vi "Save Model.vi"(7 "Group name":string, 8 "error in (no error)":errorcluster, 9 "Input onfiguration":T1={"Input File Path"=path "", "from scan..."=0, "...to scan"=0, "Lead resistance"=0.0, "Correct conductance "=FALSE, "Model parameters gap 1"={"Delta 1"=0.0, "Delta 2"=0.0, "Gama"=0.0, "Z"=0.0, "P"=0.0, "T"=0.0, "Integration range"=0.0, "Resolution"=0.0}, "Scale"=0.0, "Offset"=0.0, "Append channels"=[], "Model parameters gap 2"={"Delta 1"=0.0, "Delta 2"=0.0, "Gama"=0.0, "Z"=0.0, "P"=0.0, "T"=0.0, "Integration range"=0.0, "Resolution"=0.0}, "Gap 2 weight"=0.0, "Background conductance"=0.0, "Channels"=["V", "I", "dIdV"], "Preserve model history"=FALSE, "dIdV units"=enum."S"} {"Background conductance" step=0.0001 format="%#_6pS"; "Model parameters gap 2"."Delta 1" step=0.001 format="%#_6peV"; "Model parameters gap 2"."Resolution" format="%#_6peV"; "Model parameters gap 2"."Integration range" format="%#_6peV"; "Model parameters gap 2"."T" format="%#_6pK"; "Model parameters gap 2"."Delta 2" step=0.001 format="%#_6peV"; "Model parameters gap 2"."Gama" step=0.001 format="%#_6peV"; "Offset" scale=0.0..0.1; "Scale" scale=0.0..0.03; "Model parameters gap 1"."Delta 1" step=0.001 format="%#_6peV"; "Model parameters gap 1"."Resolution" format="%#_6peV"; "Model parameters gap 1"."Integration range" format="%#_6peV"; "Model parameters gap 1"."T" format="%#_6pK"; "Model parameters gap 1"."Delta 2" step=0.001 format="%#_6peV"; "Model parameters gap 1"."Gama" step=0.001 format="%#_6peV"; "Lead resistance" scale=0.0..80.0}, 10 "Save File Path":path, 11 "Point Contact Model in":refnum<class "Point Contact Model.lvclass">) -> (0 "error out":errorcluster, 1 "output group":string, 2 "Save File Path out":path, 3 "Point Contact Model out":refnum<class "Point Contact Model.lvclass">)   [LabVIEW 2021, in "Point Contact Model.lvclass"]
uses:
  Point Contact Model.lvclass
  Controls/PCS Config.ctl
  Parameters.ctl
  Point Contact Model.lvclass/Point Contact Model.ctl
panel:
  # "V"
  # "I"
  # "dIdV"
  # "<="
  # "<="
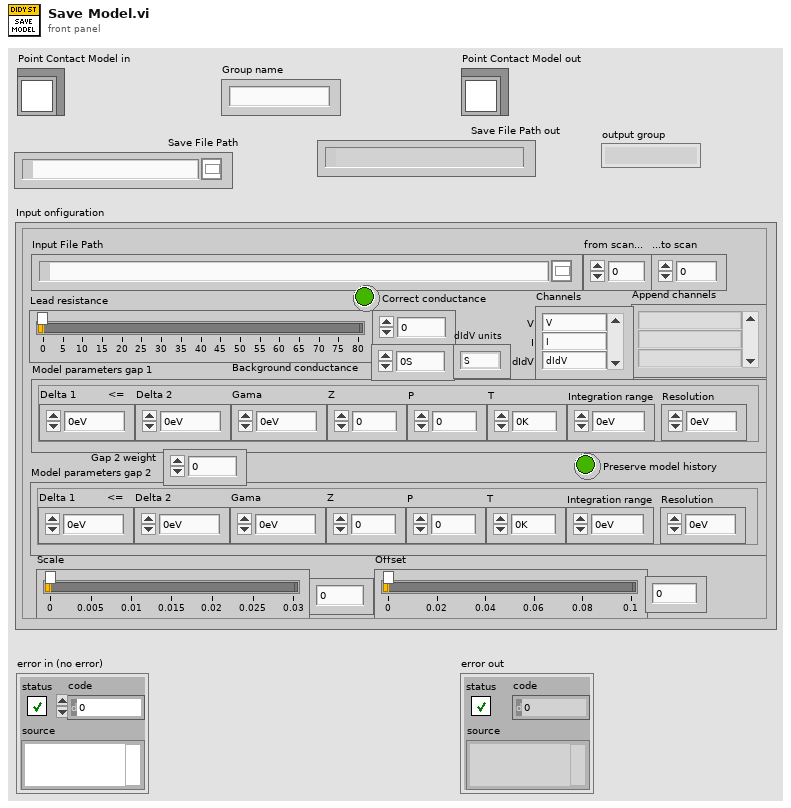
[diagram p1: front panel]
types:
  T1 = typedef "PCS Config.ctl" = cluster{"Input File Path":path, "from scan...":i32, "...to scan":i32, "Lead resistance":dbl, "Correct conductance ":bool, "Model parameters gap 1":T2, "Scale":dbl, "Offset":dbl, "Append channels":string[], "Model parameters gap 2":T2, "Gap 2 weight":dbl, "Background conductance":dbl, "Channels":string[], "Preserve model history":bool, "dIdV units":enum16{"S", "Ohm", "V"}}
  T2 = typedef "Parameters.ctl" = cluster{"Delta 1":dbl, "Delta 2":dbl, "Gama":dbl, "Z":dbl, "P":dbl, "T":dbl, "Integration range":dbl, "Resolution":dbl}
  T3 = enum16{"open", "replace", "create", "open or create", "replace or create", "replace or create with confirmation"}
  T4 = enum16{"open", "open or create", "create or replace", "create", "open (read-only)"}
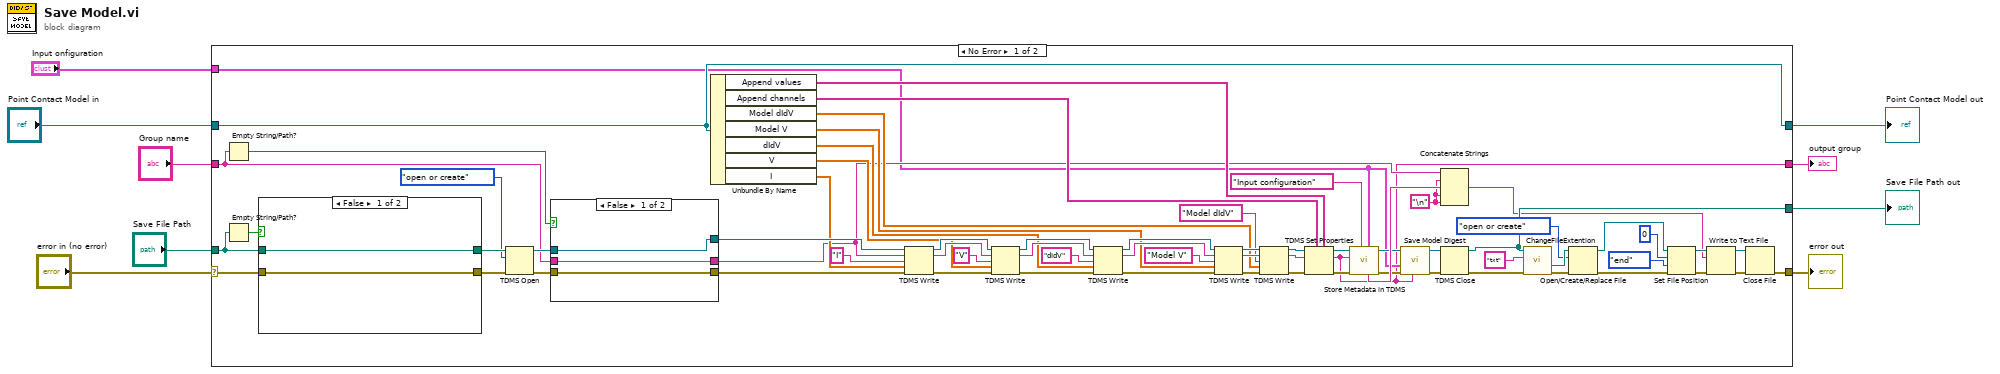
[diagram p0: block diagram]
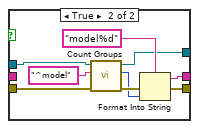
[diagram p2: hidden frame]
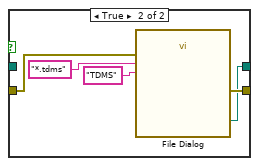
[diagram p3: hidden frame]
diagram:
  n1 = case shown="No Error" "error in (no error)" {
    selector: "error in (no error)" -> [w39 w99]
    tunnel: [w20 w99] -> w8
    tunnel: [w75 w98] -> w6
    tunnel: "Point Contact Model in" -> [w75 w98]
    tunnel: "Save File Path" -> [w76 w97]
    tunnel: [w37 w97] -> w4
    tunnel: "Input onfiguration" -> [w11 _]
    tunnel: [w10 _] -> w2
    tunnel: "Group name" -> [w16 _]
    frame No Error {
      w19 = "\n"
      n2 = Empty String/Path?(string/path=w16) -> (empty?=w17:bool)
      n3 = Empty String/Path?(string/path=w76) -> (empty?=w77:bool)
      n4 = case shown="False" w77 {
        tunnel: w39 -> [w91 w94]
        tunnel: [w91 w93] -> w72
        tunnel: [w90 w92] -> w74
        tunnel: w76 -> [w90 _]
        frame False {
        }
        frame True {
          n5 = call "File Dialog"("error in"=w94, "pattern (all files)"="*.tdms", "pattern label"="TDMS") -> ("selected path"=w92:path, "error out"=w93:errorcluster)  [unwired: 9 in, 2 out]
        }
      }
      n6 = TDMS Open(8:w72, 10:T4."open or create" ("operation (0:open)"), 11:w74) -> (0:w18:errorcluster, 3:w71:refnum<k34>)  [unwired: 4 in]
      n7 = case shown="False" w17 {
        tunnel: w71 -> [w78 w88]
        tunnel: [w79 w84] -> w70
        tunnel: [w78 w83] -> w69
        tunnel: [w80 w82] -> w27
        tunnel: w18 -> [w79 w81]
        tunnel: w16 -> [w80 _]
        frame False {
        }
        frame True {
          n8 = call "Count Groups.vi"("error in"=w81, "regular expression"="^model", "tdms file"=w88) -> ("error out"=w87:errorcluster, "Count"=w85:i32, "tdms file out"=w83:refnum<k34>)  [unwired: 5 in, 1 out]
          n9 = Format Into String(format string="model%d", error in=w87, w85) -> (resulting string=w82:string, error out=w84:errorcluster)  [unwired: 1 in]
        }
      }
      n10 = Unbundle By Name(w75) -> ("Append values"=w58:string[], "Append channels"=w59:string[], "Model dIdV"=w45:dbl[], "Model V"=w47:dbl[], "dIdV"=w56:dbl[], "V"=w64:dbl[], "I"=w55:dbl[])
      n11 = TDMS Write(0:w69, 5:w27, 7:"I", 9:w55, 11:w70) -> (4:w66:refnum<k34>, 6:w67:string, 15:w63:errorcluster)  [unwired: 1 in, 1 out]
      n12 = TDMS Write(0:w66, 5:w67, 7:"V", 9:w64, 11:w63) -> (4:w62:refnum<k34>, 6:w61:string, 15:w60:errorcluster)  [unwired: 1 in, 1 out]
      n13 = TDMS Write(0:w62, 5:w61, 7:"dIdV", 9:w56, 11:w60) -> (4:w54:refnum<k34>, 6:w50:string, 15:w52:errorcluster)  [unwired: 1 in, 1 out]
      n14 = TDMS Write(0:w54, 5:w50, 7:"Model V", 9:w47, 11:w52) -> (4:w53:refnum<k34>, 6:w49:string, 15:w51:errorcluster)  [unwired: 1 in, 1 out]
      n15 = TDMS Write(0:w53, 5:w49, 7:"Model dIdV", 9:w45, 11:w51) -> (4:w43:refnum<k34>, 6:w42:string, 15:w44:errorcluster)  [unwired: 1 in, 1 out]
      n16 = TDMS Set Properties(5:w58, 7:w59, 8:w44, 10:w42, 11:w43) -> (0:w41:errorcluster, 2:w10:string, 3:w40:refnum<k34>)  [unwired: 1 in, 1 out]
      n17 = call "Store Metadata in TDMS.vi"("Value"=w11, "name"="Input configuration", "Error In"=w41, "group name"=w10, "tdms file"=w40) -> ("Error Out"=w15:errorcluster, "tdms file out"=w13:refnum<k34>, "Meta data"=w25:string)  [unwired: 2 in, 2 out]
      n18 = call "Save Model Digest.vi"("Model group name"=w10, "error in (no error)"=w15, "Input onfiguration"=w11, "tdms file"=w13) -> ("error out"=w14:errorcluster, "tdms file out"=w12:refnum<k34>)  [unwired: 5 in, 1 out]
      n19 = Concatenate Strings(w27, w19, w25, w19, w19) -> (w26:string)
      n20 = TDMS Close(8:w14, 11:w12) -> (0:w35:errorcluster, 3:w37:path)
      n21 = call "ChangeFileExtention.vi"("Error In"=w35, "New extension"="txt", "File Path"=w37) -> ("Error Out"=w21:errorcluster, "Path with new extension"=w34:path)  [unwired: 3 in, 4 out]
      n22 = Open/Create/Replace File(file path (use dialog)=w34, error in=w21, operation (0:open)=T3."open or create") -> (refnum out=w32:refnum<file>, error out=w29:errorcluster)  [unwired: 3 in, 1 out]
      n23 = Set File Position(offset (in bytes) (0)=i64 0, refnum=w32, from (0:start)=enum16{"start", "end", "current"}."end", error in=w29) -> (refnum out=w28:refnum<file>, error out=w24:errorcluster)
      n24 = Write to Text File(file (use dialog)=w28, text=w26, error in=w24) -> (refnum out=w23:refnum<file>, error out=w22:errorcluster)  [unwired: 1 in, 1 out]
      n25 = Close File(refnum=w23, error in=w22) -> (error out=w20:errorcluster)  [unwired: 1 out]
    }
    frame Error {
    }
  }
  "error out" <- w8
  "Point Contact Model out" <- w6
  "Save File Path out" <- w4
  "output group" <- w2
